vi "Legend Bar Prefix.vi"() -> (2 "Prefix Out":string)   [LabVIEW 2017, in "3D Bar.lvclass"]
uses:
  <vilib>/Math Plots/3D Math Plots/3D Bar/3D Bar/3D Bar.lvclass
panel:
  in  "Prefix":string="Bar"
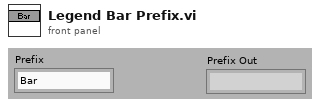
[diagram p1: front panel]
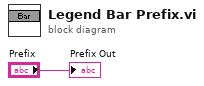
[diagram p0: block diagram]
diagram:
  "Prefix Out" <- "Prefix"
